vi "Test PWM FGV.vi"() -> ()   [LabVIEW 2013]
doc: "This sub-VI tests the PWM functional global variable and can be used to aid in setting up communication\nwith motors."
uses:
  Controls/table_axis_enum.ctl
  Controls/PWM_test_ctrl_cluster.ctl
  Controls/PWM_data_cluster.ctl
  Controls/PWM_state_enum.ctl
  <vilib>/DAQmx/write.llb/DAQmx Write (Digital Bool 1Line 1Point).vi
  <vilib>/DAQmx/write.llb/DAQmx Write (Digital 1D Bool NChan 1Samp 1Line).vi
  <vilib>/DAQmx/miscellaneous.llb/DAQmx Fill In Error Info.vi
panel:
  in  "Motor Test Controls":T1
  in  "Axis Enum":T2
  in  "PWM Duty Cycle":dbl(knob) min=0.0 max=100.0 step=1.0 scale=0.0..100.0
  in  "Stop Button":bool
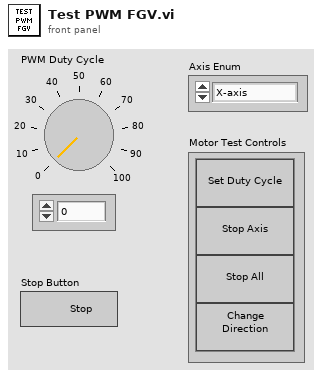
[diagram p1: front panel]
types:
  T1 = typedef "PWM_test_ctrl_cluster.ctl" = cluster{"Set Speed":bool, "Stop Axis":bool, "Stop All":bool, "Change Dir":bool}
  T2 = typedef "table_axis_enum.ctl" = enum16{"X-axis", "Y-axis", "Z-axis", "W-axis"}
  T3 = typedef "PWM_data_cluster.ctl" = cluster{"frequency":dbl, "Duty Cycle (%)":dbl, "Axis Enum":T2, "Function Enum":T4}
  T4 = typedef "PWM_state_enum.ctl" = enum16{"Initialize", "SetAxisSpeed", "StopAxis", "StopAll", "Shutdown"}
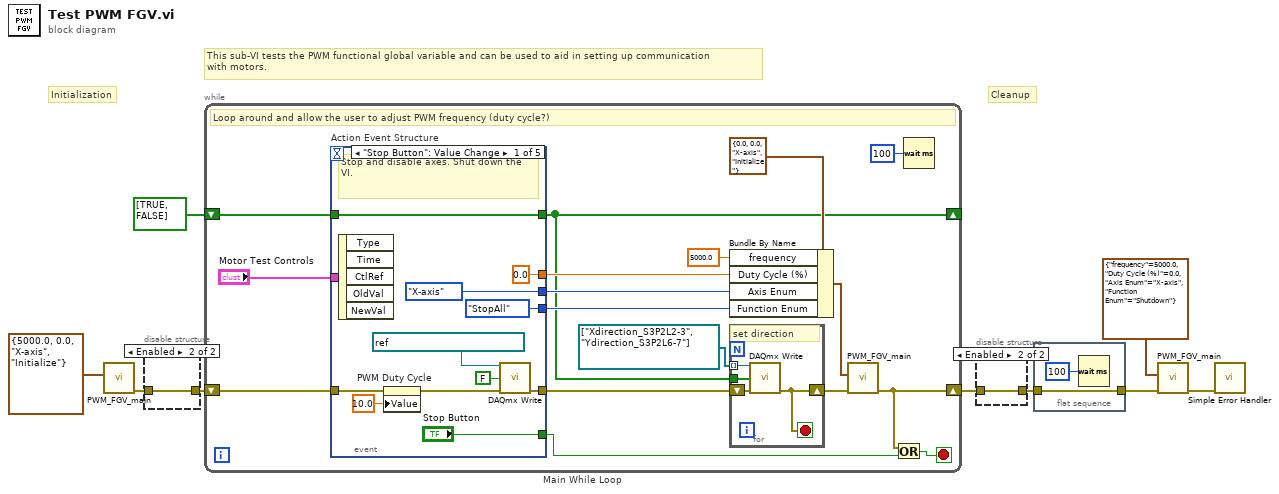
[diagram p0: block diagram]
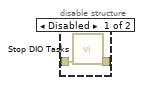
[diagram p2: hidden frame]
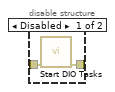
[diagram p3: hidden frame]
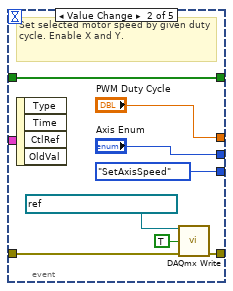
[diagram p4: hidden frame]
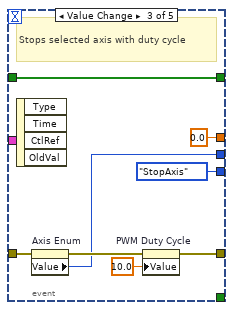
[diagram p5: hidden frame]
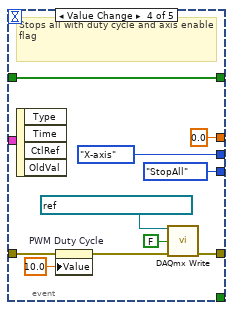
[diagram p6: hidden frame]
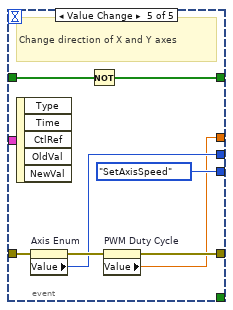
[diagram p7: hidden frame]
diagram:
  # "Cleanup"
  # "Initialization"
  # "This sub-VI tests the PWM functional global variable and can be used to aid in setting up communication\nwith motors."
  n1 = call "PWM_FGV_main.vi"("PWM FGV Data"=T3 {"frequency"=5000.0, "Duty Cycle (%)"=0.0, "Axis Enum"=enum."X-axis", "Function Enum"=enum."Initialize"}) -> ("Error Out"=w5:errorcluster)  [unwired: 10 in]
  n2 = disable-structure shown="Enabled" {
    disable-tunnel: w5 -> [w11 w12]
    disable-tunnel: [w10 w12] -> w4
    frame Disabled {
      n3 = call "Start DIO Tasks.vi"("error in (no error)"=w11) -> ("error out"=w10:errorcluster)  [unwired: 10 in]
    }
    frame Enabled {
    }
  }
  n4 = while "Main While Loop" {
    shift-right: [w28] -> w6
    shift-left: w4 -> [w19]
    shift-right: [w14] -> _
    shift-left: bool[] [TRUE, FALSE] -> [w15]
    stop <- w29 stop-if-true
    # "Loop around and allow the user to adjust PWM frequency (duty cycle?)"
    n5 = event "Action Event Structure" shown="[0] \"Stop Button\": Value Change" {
      selector: _ -> [_ _ _ _ _]
      dyn-events: _ -> [_ _ _ _ _]
      timeout: _ -> [_ _ _ _ _]
      tunnel: [0.0 ("PWM Duty Cycle") "PWM Duty Cycle" 0.0 ("PWM Duty Cycle") 0.0 ("PWM Duty Cycle") w73] -> w23
      tunnel: "Motor Test Controls" -> [_ _ _ _ _]
      tunnel: [table_axis_enum."X-axis" ("Axis Enum") "Axis Enum" w53 table_axis_enum."X-axis" ("Axis Enum") w74] -> w21
      tunnel: [PWM_state_enum."StopAll" ("Function Enum") PWM_state_enum."SetAxisSpeed" ("Function Enum") PWM_state_enum."StopAxis" ("Function Enum") PWM_state_enum."StopAll" ("Function Enum") PWM_state_enum."SetAxisSpeed" ("Function Enum")] -> w20
      tunnel: w19 -> [w36 w46 w55 w62 w77]
      tunnel: [w39 w50 w56 w67 w75] -> w18
      tunnel: ["Stop Button" _ _ _ _] -> w17
      tunnel: w15 -> [w40 w47 w58 w64 w72]
      tunnel: [w40 w47 w58 w64 w71] -> w14
      event "Stop Button": Value Change {
        # "Stop and disable axes. Shut down the VI."
        n6 = event-data() -> ()  [unwired: 1 in, 5 out]
        n7 = property on="PWM Duty Cycle" class="Knob (strict)"(error in=w36, "Value"=10.0 ("PWM Duty Cycle")) -> (error out=w35:errorcluster)  [unwired: 1 in, 1 out]
        n8 = call-poly <vilib>:"DAQmx Write.vi"("task/channels in"=refnum<k21> "XYmotorEnable_S3P2L1", "data"=FALSE, "error in"=w35) -> ("error out"=w39:errorcluster)  [unwired: 10 in, 2 out]
      }
      event Value Change {
        # "Set selected motor speed by given duty cycle. Enable X and Y."
        n9 = event-data() -> ()  [unwired: 1 in, 4 out]
        n10 = call-poly <vilib>:"DAQmx Write.vi"("task/channels in"=refnum<k21> "XYmotorEnable_S3P2L1", "data"=TRUE, "error in"=w46) -> ("error out"=w50:errorcluster)  [unwired: 10 in, 2 out]
      }
      event Value Change {
        # "Stops selected axis with duty cycle"
        n11 = event-data() -> ()  [unwired: 1 in, 4 out]
        n12 = property on="Axis Enum" class="Enum (strict)"(error in=w55) -> (error out=w54:errorcluster, "Value"=w53:T2)  [unwired: 1 in, 1 out]
        n13 = property on="PWM Duty Cycle" class="Knob (strict)"(error in=w54, "Value"=10.0 ("PWM Duty Cycle")) -> (error out=w56:errorcluster)  [unwired: 1 in, 1 out]
      }
      event Value Change {
        # "Stops all with duty cycle and axis enable flag"
        n14 = event-data() -> ()  [unwired: 1 in, 4 out]
        n15 = property on="PWM Duty Cycle" class="Knob (strict)"(error in=w62, "Value"=10.0 ("PWM Duty Cycle")) -> (error out=w61:errorcluster)  [unwired: 1 in, 1 out]
        n16 = call-poly <vilib>:"DAQmx Write.vi"("task/channels in"=refnum<k21> "XYmotorEnable_S3P2L1", "data"=FALSE, "error in"=w61) -> ("error out"=w67:errorcluster)  [unwired: 10 in, 2 out]
      }
      event Value Change {
        # "Change direction of X and Y axes"
        n17 = event-data() -> ()  [unwired: 1 in, 5 out]
        n18 = property on="Axis Enum" class="Enum (strict)"(error in=w77) -> (error out=w76:errorcluster, "Value"=w74:T2)  [unwired: 1 in, 1 out]
        n19 = Not(x=w72) -> (.not. x?=w71:bool[])
        n20 = property on="PWM Duty Cycle" class="Knob (strict)"(error in=w76) -> (error out=w75:errorcluster, "Value"=w73:dbl)  [unwired: 1 in, 1 out]
      }
    }
    n21 = Bundle By Name(cluster=T3 {"frequency"=0.0, "Duty Cycle (%)"=0.0, "Axis Enum"=enum."X-axis", "Function Enum"=enum."Initialize"} ("PWM FGV Data"), "frequency"=5000.0, "Duty Cycle (%)"=w23, "Axis Enum"=w21, "Function Enum"=w20) -> (w26:T3)
    n22 = for {
      tunnel: w14 -> [w32]
      shift-right: [w31] -> w16
      shift-left: w18 -> [w33]
      tunnel: refnum<k21>[] ["Xdirection_S3P2L2-3", "Ydirection_S3P2L6-7"] -> [w30] mode=indexing
      stop <- w31 stop-if-true
      # "set direction"
      n23 = call-poly <vilib>:"DAQmx Write.vi"("task/channels in"=w30, "data"=w32, "error in"=w33) -> ("error out"=w31:errorcluster)  [unwired: 10 in, 2 out]
    }
    n24 = call "PWM_FGV_main.vi"("Error In"=w16, "PWM FGV Data"=w26) -> ("Error Out"=w28:errorcluster)  [unwired: 9 in]
    n25 = Or(x=w28, y=w17) -> (x .or. y?=w29:bool)
    n26 = Wait (ms)(milliseconds to wait=u32 100) -> ()  [unwired: 1 out]
  }
  n27 = disable-structure shown="Enabled" {
    disable-tunnel: w6 -> [w80 w81]
    disable-tunnel: [w79 w81] -> w2
    frame Disabled {
      n28 = call "Stop DIO Tasks.vi"("Error In"=w80) -> ("error out"=w79:errorcluster)  [unwired: 10 in]
    }
    frame Enabled {
    }
  }
  n29 = flat-sequence {
    tunnel: w2 -> [w83]
    tunnel: [w83] -> w1
    frame #0 {
      n30 = Wait (ms)(milliseconds to wait=u32 100) -> ()  [unwired: 1 out]
    }
  }
  n31 = call "PWM_FGV_main.vi"("Error In"=w1, "PWM FGV Data"=T3 {"frequency"=5000.0, "Duty Cycle (%)"=0.0, "Axis Enum"=enum."X-axis", "Function Enum"=enum."Shutdown"}) -> ("Error Out"=w7:errorcluster)  [unwired: 9 in]
  n32 = call <vilib>:"Simple Error Handler.vi"("error in (no error)"=w7) -> ()  [unwired: 4 in, 5 out]
